vi "BRig_Host__Loop_Producer__tcp_System__Data_storeFiles_buildMessage.vi"(6 "input_n":i32, 9 "input_stored":bool[](array[boolean]), 10 "input_exist_source":bool[](array[boolean]), 11 "input_arrFilenames":string[](array[string])) -> (0 "output_msg":string)   [LabVIEW 2014]
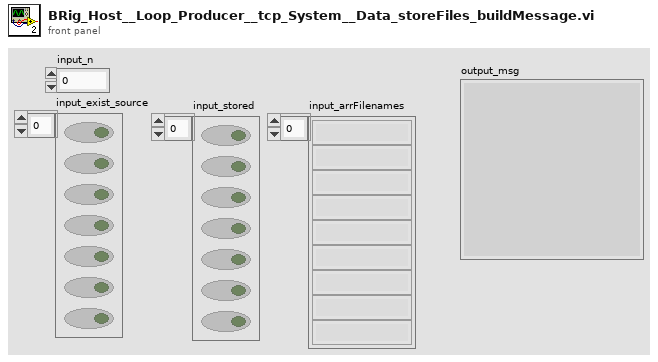
[diagram p1: front panel]
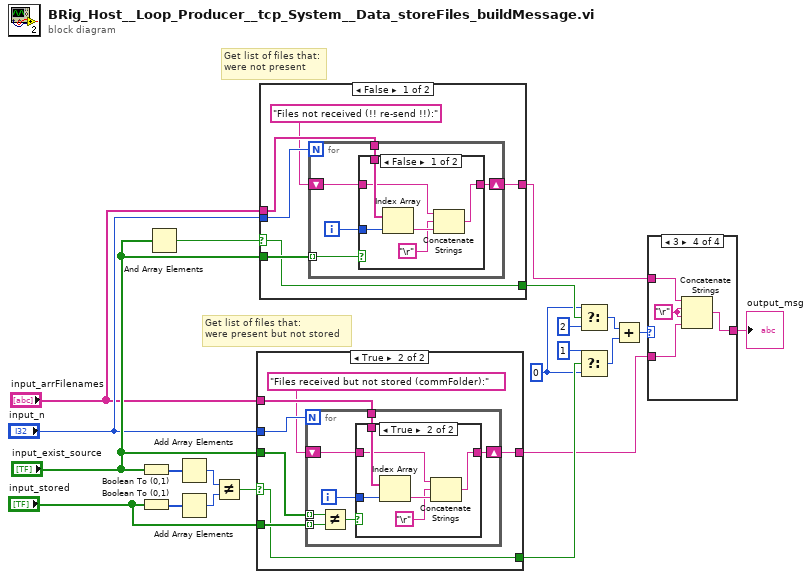
[diagram p0: block diagram]
diagram:
  w1 = u8 0
  # "Get list of files that:\nwere present but not stored"
  # "Get list of files that:\nwere not present"
  n1 = Boolean To (0,1)(Boolean="input_exist_source") -> (0, 1=w21:i16[])
  n2 = Boolean To (0,1)(Boolean="input_stored") -> (0, 1=w20:i16[])
  n3 = And Array Elements(Boolean array="input_exist_source") -> (logical AND=w15:bool)
  n4 = Add Array Elements(numeric array=w21) -> (sum=w19:i16)
  n5 = Add Array Elements(numeric array=w20) -> (sum=w18:i16)
  n6 = Not Equal?(x=w19, y=w18) -> (x != y?=w17:bool)
  n7 = case shown="True" w17 {
    selector: w17 -> [w22 w23]
    tunnel: "input_exist_source" -> [_ w28]
    tunnel: "input_stored" -> [_ w27]
    tunnel: "input_n" -> [_ w29]
    tunnel: "input_arrFilenames" -> [_ w26]
    tunnel: [_ w24] -> w7
    tunnel: [w22 w23] -> w11
    frame False {
    }
    frame True {
      n8 = for {
        N: w29 -> [_]
        tunnel: w28 -> [w35] mode=indexing
        tunnel: w27 -> [w36] mode=indexing
        tunnel: w26 -> [w33]
        shift-right: [w30] -> w24
        shift-left: "Files received but not stored (commFolder):" -> [w31]
        i -> [w32]
        n9 = Not Equal?(x=w35, y=w36) -> (x != y?=w34:bool)
        n10 = case shown="True" w34 {
          tunnel: w33 -> [_ w43]
          tunnel: w32 -> [_ w42]
          tunnel: w31 -> [w37 w39]
          tunnel: [w37 w38] -> w30
          frame False {
          }
          frame True {
            n11 = Index Array(array=w43, index=w42) -> (element=w41:string)
            n12 = Concatenate Strings(w39, "\r", w41) -> (w38:string)
          }
        }
      }
    }
  }
  n13 = case shown="False" w15 {
    selector: w15 -> [w44 w62]
    tunnel: "input_exist_source" -> [w48 _]
    tunnel: "input_n" -> [w49 _]
    tunnel: "input_arrFilenames" -> [w47 _]
    tunnel: [w45 _] -> w8
    tunnel: [w44 w62] -> w10
    frame False {
      n14 = for {
        N: w49 -> [_]
        tunnel: w48 -> [w50] mode=indexing
        tunnel: w47 -> [w54]
        shift-right: [w51] -> w45
        shift-left: "Files not received (!! re-send !!):" -> [w52]
        i -> [w53]
        n15 = case shown="False" w50 {
          tunnel: w54 -> [w60 _]
          tunnel: w53 -> [w59 _]
          tunnel: w52 -> [w56 w61]
          tunnel: [w55 w61] -> w51
          frame False {
            n16 = Index Array(array=w60, index=w59) -> (element=w58:string)
            n17 = Concatenate Strings(w56, "\r", w58) -> (w55:string)
          }
          frame True {
          }
        }
      }
    }
    frame True {
    }
  }
  n18 = Select(t=w1, s=w10, f=u8 2) -> (s? t:f=w5:u8)
  n19 = Select(t=u8 1, s=w11, f=w1) -> (s? t:f=w4:u8)
  n20 = Add(x=w5, y=w4) -> (x+y=w6:u8)
  n21 = case shown="3" w6 {
    tunnel: w8 -> [_ _ w64 w68]
    tunnel: w7 -> [_ w63 _ w66]
    tunnel: [_ w63 w64 w65] -> w3
    frame 0, Default {
    }
    frame 1 {
    }
    frame 2 {
    }
    frame 3 {
      w67 = "\r"
      n22 = Concatenate Strings(w68, w67, w67, w66) -> (w65:string)
    }
  }
  "output_msg" <- w3
